vi "Compute Registry Key.vi"(10 "SMO GUID":string, 11 "Registry's SecretKey":string) -> (3 "Registry Key":string)   [LabVIEW 2013, in "Registry-SMO.lvclass"]
uses:
  Registry-SMO.lvclass
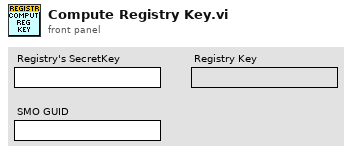
[diagram p1: front panel]
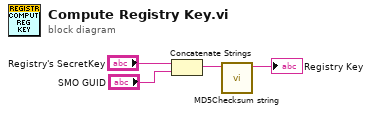
[diagram p0: block diagram]
diagram:
  n1 = Concatenate Strings("Registry's SecretKey", "SMO GUID") -> (w1:string)
  n2 = call <vilib>:"MD5Checksum string.vi"("Message String"=w1) -> ("MD5 message-digest"=→"Registry Key":string)  [unwired: 10 in]
